vi "example-RaiseErrorIf.vi"() -> ()   [LabVIEW 2019]
panel:
  out "error out":errorcluster
  in  "error in (no error)":errorcluster
  in  "String":string
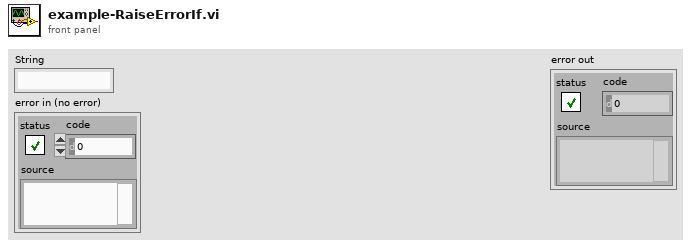
[diagram p1: front panel]
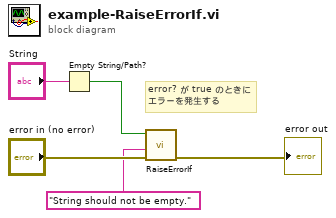
[diagram p0: block diagram]
diagram:
  # "error? が true のときに\nエラーを発生する"
  n1 = Empty String/Path?(string/path="String") -> (empty?=w2:bool)
  n2 = call "RaiseErrorIf.vi"("error in (no error)"="error in (no error)", "error message"="String should not be empty." ("String"), "error? (true)"=w2) -> ("error out"=→"error out":errorcluster)  [unwired: 8 in]
